vi "Read Channel Configuration.vi"(8 "error in (no error)":errorcluster, 11 "Software Lock-in in":refnum<class "Software Lock-in.lvclass">) -> (0 "error out":errorcluster, 3 "Software Lock-in out":refnum<class "Software Lock-in.lvclass">)   [LabVIEW 2016, in "Software Lock-in.lvclass"]
uses:
  Software Lock-in.lvclass
  Software Lock-in.lvclass/Software Lock-in.ctl
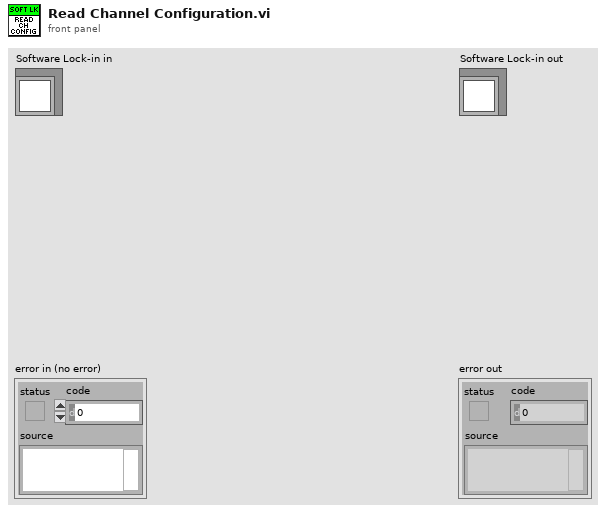
[diagram p1: front panel]
types:
  T1 = typedef "Lockin Parameters.ctl" = cluster{"Frequency":dbl, "Phase":dbl, "Syncronous":bool, "Points per sine wave":i32, "DDS":bool, "Frequency word":u32, "Phase word":u32, "DDS modulus":i64, "DDS clock":dbl}
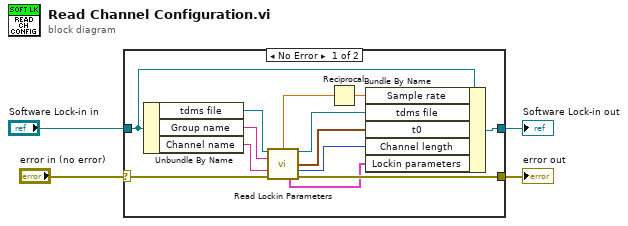
[diagram p0: block diagram]
diagram:
  n1 = case shown="No Error" "error in (no error)" {
    selector: "error in (no error)" -> [w14 w19]
    tunnel: [w13 w19] -> w3
    tunnel: [w15 w18] -> w1
    tunnel: "Software Lock-in in" -> [w17 w18]
    frame No Error {
      n2 = Unbundle By Name(w17) -> ("tdms file"=w16:refnum<k34>, "Group name"=w12:string, "Channel name"=w11:string)
      n3 = call "Read Lockin Parameters.vi"("tdms file"=w16, "group name in"=w12, "Channel name"=w11, "Error In"=w14) -> ("dt"=w6:dbl, "tdms file out"=w7:refnum<k34>, "t0"=w10:timestamp, "Channel length"=w9:u64, "Lockin parameters out"=w8:T1, "Error Out"=w13:errorcluster)  [unwired: 6 in]
      n4 = Reciprocal(x=w6) -> (1/x=w5:dbl)
      n5 = Bundle By Name(cluster=w17, "Sample rate"=w5, "tdms file"=w7, "t0"=w10, "Channel length"=w9, "Lockin parameters"=w8) -> (w15:refnum<class "Software Lock-in.lvclass">)
    }
    frame Error {
    }
  }
  "error out" <- w3
  "Software Lock-in out" <- w1
